vi "PH_ImageCalibrator.calibration data file.vi"(2 "Camera Instance":string, 5 "error in":errorcluster) -> (17 "File to save Cam Calibration Data in":path, 19 "error out":errorcluster)   [LabVIEW 2014, in "PH_ImageCalibrator.lvlib"]
doc: "This VI is forseen to be used in the save data file VI as well as in VIs used to read data from hard disk. If all inputs are connected, this VI creates a file name."
uses:
  PH_ImageCalibrator.lvlib
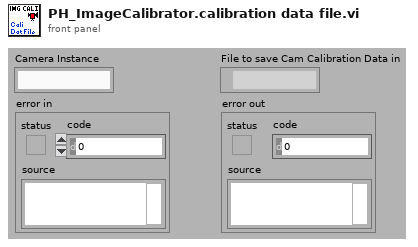
[diagram p1: front panel]
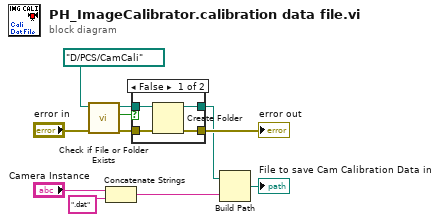
[diagram p0: block diagram]
diagram:
  n1 = call <vilib>:"Check if File or Folder Exists.vi"("error in (no error)"="error in", "path"=path "D:/PCS/CamCali" ("base path")) -> ("error out"=w4:errorcluster, "file or folder exists?"=w6:bool, "dup path"=w3:path)  [unwired: 7 in]
  n2 = Concatenate Strings("Camera Instance", ".dat" ("string")) -> (w11:string)
  n3 = case shown="False" w6 {
    tunnel: w4 -> [w14 w16]
    tunnel: w3 -> [w15 w17]
    tunnel: [w12 w17] -> w2
    tunnel: [w13 w16] -> w8
    frame False {
      n4 = Create Folder(path (use dialog)=w15, error in=w14) -> (created path=w12:path, error out=w13:errorcluster)  [unwired: 1 in, 1 out]
    }
    frame True {
    }
  }
  "error out" <- w8
  n5 = Build Path(base path=w2, name or relative path=w11) -> (appended path=→"File to save Cam Calibration Data in":path)
